vi "Step Type Menu Item.vi"(10 "Group (From Step)":string, 11 "Step Type Name":string) -> (0 "error out":errorcluster, 3 "StepTypeMenuItem":refnum<class "StepTypeMenuItem.lvclass">)   [LabVIEW 2020, in "TSnax UI.lvlib" / "InsertionPalettePanel.lvclass"]
uses:
  InsertionPalettePanel.lvclass
  StepTypeMenuItem/StepTypeMenuItem.lvclass
  TSnax/Common StepType Subproperties.ctl
  b736253d-652d-475f-9fd0-7b127d7733e5.vi
  4a5c9662-0516-4c52-87d6-6fa9d900fcf8.vi
  b736253d-652d-475f-9fd0-7b127d7733e5.vi/cb391dcb-11b9-4fdf-8aeb-34376e1cbb94.vi
  b736253d-652d-475f-9fd0-7b127d7733e5.vi/d46dfaf5-493f-4f70-8e7b-742c39259470.vi
  b736253d-652d-475f-9fd0-7b127d7733e5.vi/d46dfaf5-493f-4f70-8e7b-742c39259470.vi/5752542f-8fd2-4c21-a269-ab70273be737.vi
  TSnax/PropertyObject/Get Val STR.vi
  TSnax/PropertyObject/Eval Expression String.vi
  TSnax/PropertyObject/PropertyObject.lvclass
  InsertionPalettePanel.lvclass/InsertionPalettePanel.ctl
  TSnax/Engine/Engine.lvclass
  TSnax/TSnax.lvlib
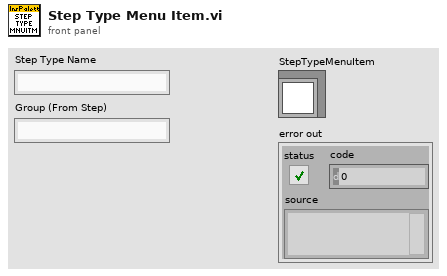
[diagram p1: front panel]
types:
  T1 = typedef "TSnax.lvlib/Common StepType Subproperties.ctl" = enum16{"AppliesToBlockStructure", "BlockEndTypes", "BlockStartTypes", "CanEncapsulate", "Category", "DefaultNameFormat", "DescriptionFormat", "Menu.Category", "Menu.Group", "Menu.ItemName", "Substeps.OnNewStep", "Substeps.Edit"}
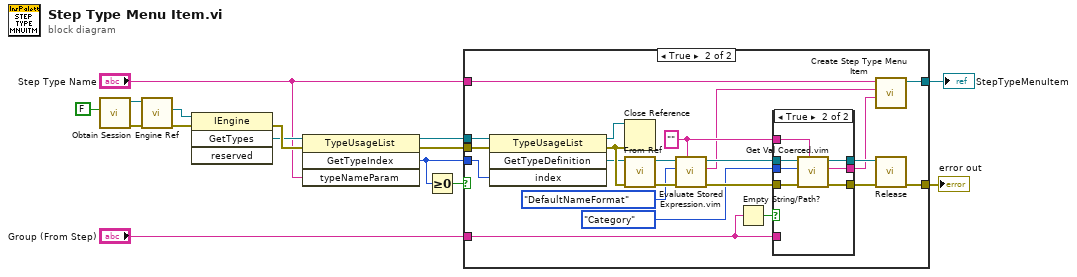
[diagram p0: block diagram]
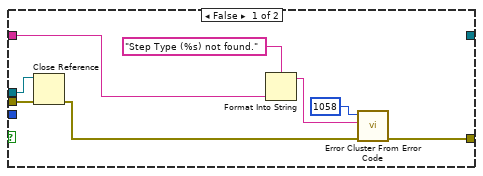
[diagram p2: hidden frame]
diagram:
  n1 = call "Obtain Session.vi"("Create if needed? (T)"=FALSE) -> ("error out"=w12:errorcluster, "Engine out"=w13:refnum<class "Engine.lvclass">)  [unwired: 9 in]
  n2 = call "Engine Ref.vi"("error in (no error)"=w12, "Engine in"=w13) -> ("error out"=w9:errorcluster, "Engine"=w11:refnum<k7>)  [unwired: 7 in, 1 out]
  n3 = invoke class="IEngine" method="GetTypes"(reference=w11, error in=w9) -> (error out=w15:errorcluster, "GetTypes"=w10:refnum<k7>)  [unwired: 2 in, 2 out]
  n4 = invoke class="TypeUsageList" method="GetTypeIndex"(reference=w10, error in=w15, "typeNameParam"="Step Type Name") -> (reference out=w5:refnum<k7>, error out=w8:errorcluster, "GetTypeIndex"=w6:i32)  [unwired: 1 in, 1 out]
  n5 = Greater Or Equal To 0?(x=w6) -> (x >= 0?=w7:bool)
  n6 = case shown="True" w7 {
    tunnel: w8 -> [w22 w42]
    tunnel: w6 -> [_ w41]
    tunnel: w5 -> [w21 w43]
    tunnel: "Group (From Step)" -> [_ w30]
    tunnel: "Step Type Name" -> [w17 w35]
    tunnel: [_ w25] -> w2
    tunnel: [w19 w24] -> w1
    frame False {
      n7 = Close Reference(reference=w21, error in (no error)=w22) -> (error out=w20:errorcluster)
      n8 = Format Into String(format string="Step Type (%s) not found.", w17) -> (resulting string=w16:string)  [unwired: 2 in, 1 out]
      n9 = call <vilib>:"Error Cluster From Error Code.vi"("error in (no error)"=w20, "error message (\"\")"=w16, "error code (0)"=1058) -> ("error out"=w19:errorcluster)  [unwired: 6 in]
    }
    frame True {
      w33 = ""
      n10 = invoke class="TypeUsageList" method="GetTypeDefinition"(reference=w43, error in=w42, "index"=w41) -> (reference out=w39:refnum<k7>, error out=w44:errorcluster, "GetTypeDefinition"=w40:refnum<k7>)  [unwired: 1 in, 1 out]
      n11 = Close Reference(reference=w39, error in (no error)=w44) -> ()  [unwired: 1 out]
      n12 = call "From Ref.vi"("error in (no error)"=w44, "PropertyObject"=w40) -> ("error out"=w37:errorcluster, "PropertyObject out"=w38:refnum<class "PropertyObject.lvclass">)  [unwired: 8 in]
      n13 = call "Evaluate Stored Expression.vim"("Result Type (PropertyObject)"=w33, "error in (no error)"=w37, "Lookup String (Self)"=Common_StepType_Subproperties."DefaultNameFormat" ("Common StepType Subproperties"), "PropertyObject in"=w38) -> ("error out"=w45:errorcluster, "Result"=w31:string, "PropertyObject out"=w34:refnum<class "PropertyObject.lvclass">)  [unwired: 5 in]
      n14 = Empty String/Path?(string/path=w30) -> (empty?=w29:bool)
      n15 = case shown="True" w29 {
        tunnel: w45 -> [w47 w55]
        tunnel: w34 -> [w48 w54]
        tunnel: w33 -> [_ w53]
        tunnel: Common_StepType_Subproperties."Category" ("Common StepType Subproperties") -> [_ w52]
        tunnel: w30 -> [w46 _]
        tunnel: [w46 w51] -> w26
        tunnel: [w47 w50] -> w27
        tunnel: [w48 w49] -> w28
        frame False {
        }
        frame True {
          n16 = call "Get Val Coerced.vim"("Value Type (String)"=w53, "error in (no error)"=w55, "Lookup String"=w52, "PropertyObject in"=w54) -> ("error out"=w50:errorcluster, "Value"=w51:string, "PropertyObject out"=w49:refnum<class "PropertyObject.lvclass">)  [unwired: 5 in]
        }
      }
      n17 = call "Create Step Type Menu Item.vi"("Group"=w26, "Display Name"=w31, "Step Type"=w35) -> ("Step Type Menu Item"=w25:refnum<class "StepTypeMenuItem.lvclass">)  [unwired: 8 in]
      n18 = call-dynamic "Release.vi"("error in (no error)"=w27, "PropertyObject in"=w28) -> ("error out"=w24:errorcluster)  [unwired: 9 in]
    }
  }
  "StepTypeMenuItem" <- w2
  "error out" <- w1
